vi "Serial Log.vi"(7 "State":enum16{"Init", "Write", "Read"}(ring), 8 "error in (no error)":errorcluster, 11 "String":string) -> (0 "error out":errorcluster, 2 "Big String":string, 3 "Logs":string[](array[string]))   [LabVIEW 2011]
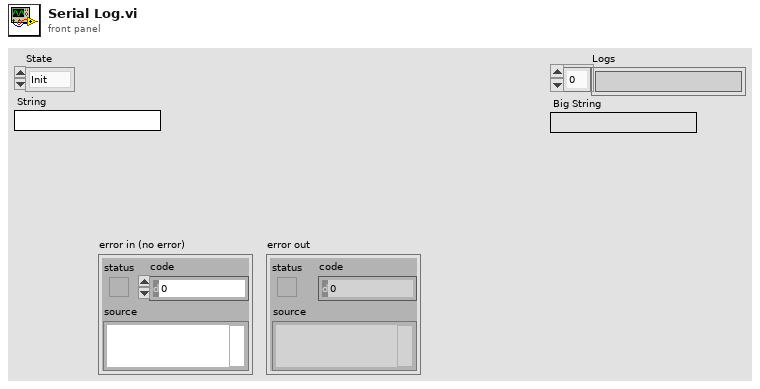
[diagram p1: front panel]
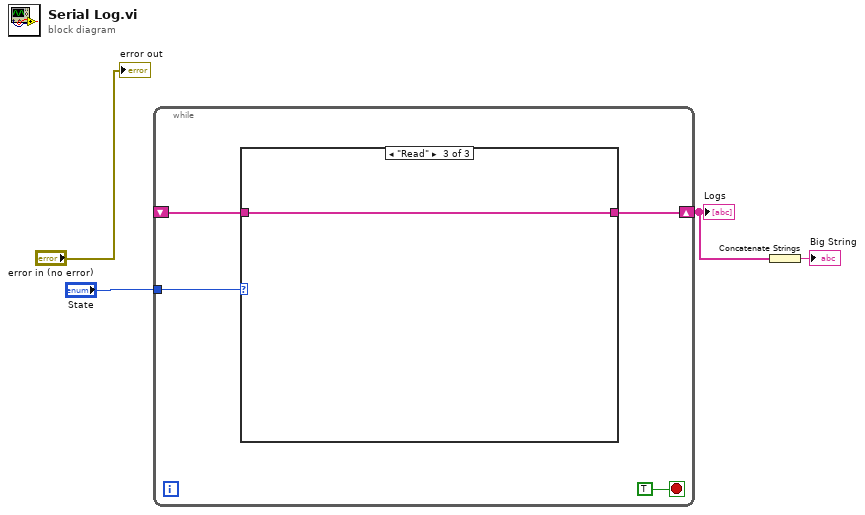
[diagram p0: block diagram]
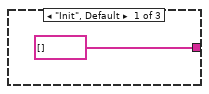
[diagram p2: hidden frame]
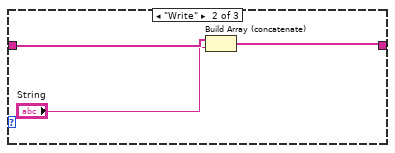
[diagram p3: hidden frame]
diagram:
  n1 = while {
    tunnel: "State" -> [w8]
    shift-right: [w7] -> w3
    shift-left: _ -> [w6]
    stop <- TRUE stop-if-true
    n2 = case shown="\"Read\"" w8 {
      tunnel: [string[] [] w11 w13] -> w7
      tunnel: w6 -> [_ w12 w13]
      frame "Init", Default {
      }
      frame "Write" {
        n3 = Build Array (concatenate)(w12, "String") -> (w11:string[])
      }
      frame "Read" {
      }
    }
  }
  "Logs" <- w3
  n4 = Concatenate Strings(w3) -> (→"Big String":string)
  "error out" <- "error in (no error)"
